vi "Convert Variant to NT Cluster.vi"(11 "NewVal":variant) -> (3 "Field Value":T1)   [LabVIEW 2017]
doc: "Attempt to convert the LV variant type to the various NT types. If not able to do so, it may be stored as a serialized variant or become an invalid NT v ariable."
uses:
  <vilib>/Rock Robotics/Network Tables/Field Data.ctl
  <vilib>/Rock Robotics/Network Tables/Field Type.ctl
  <vilib>/Rock Robotics/Network Tables/Sequence.ctl
panel:
  out "type string":i16[](array[numeric]) format="%.0x"
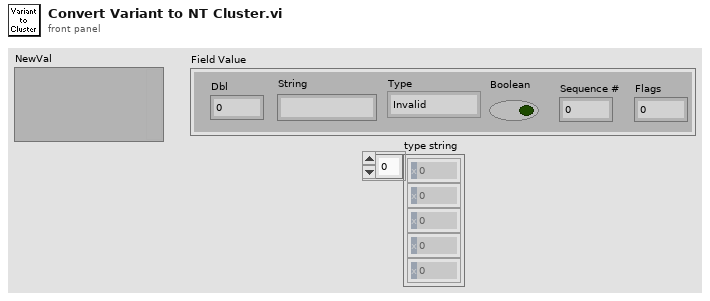
[diagram p1: front panel]
types:
  T1 = typedef "Field Data.ctl" = cluster{"Dbl":dbl, "String":string, "Type":T2, "Boolean":bool, "Sequence #":T3, "Flags":u8}
  T2 = typedef "Field Type.ctl" = enum8{"Invalid", "Bool", "Numeric", "String", "Raw", "Boolean Array", "Numeric Array", "String Array", "RPC"}
  T3 = typedef "Sequence.ctl" = u16
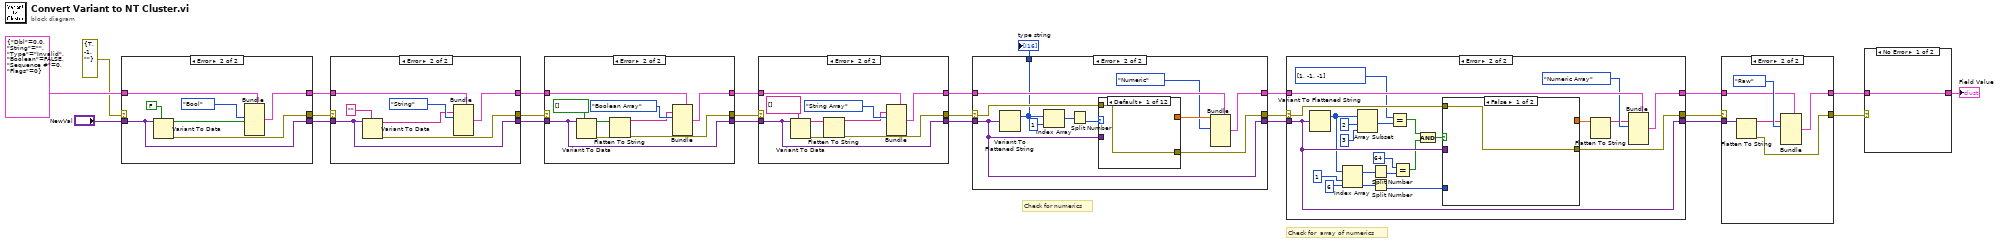
[diagram p0: block diagram]
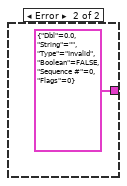
[diagram p3: hidden frame]
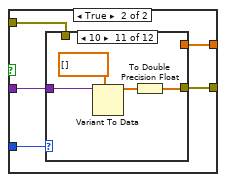
[diagram p5: hidden frame]
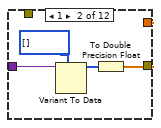
[diagram p7: hidden frame]
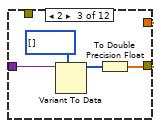
[diagram p8: hidden frame]
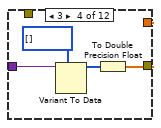
[diagram p9: hidden frame]
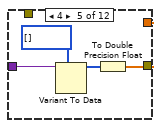
[diagram p10: hidden frame]
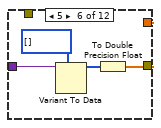
[diagram p11: hidden frame]
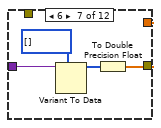
[diagram p12: hidden frame]
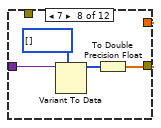
[diagram p13: hidden frame]
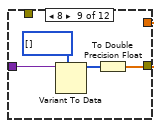
[diagram p14: hidden frame]
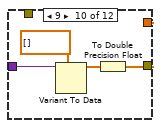
[diagram p15: hidden frame]
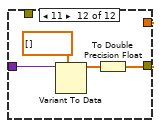
[diagram p16: hidden frame]
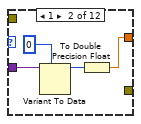
[diagram p18: hidden frame]
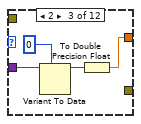
[diagram p19: hidden frame]
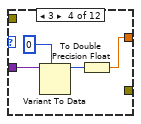
[diagram p20: hidden frame]
diagram:
  # "Check for  array of numerics"
  # "Check for numerics"
  n1 = case shown="Error" errorcluster {"status"=TRUE, "code"=-1, "source"=""} ("error constant") {
    selector: errorcluster {"status"=TRUE, "code"=-1, "source"=""} ("error constant") -> [w27 _]
    tunnel: "NewVal" -> [w26 w31]
    tunnel: T1 {"Dbl"=0.0, "String"="", "Type"=enum."Invalid", "Boolean"=FALSE, "Sequence #"=0, "Flags"=0} ("Field Value") -> [w28 w35]
    tunnel: [w28 w32] -> w19
    tunnel: [w27 w33] -> w18
    tunnel: [w26 w31] -> w17
    frame No Error {
    }
    frame Error {
      n2 = Variant To Data(type=FALSE ("status"), Variant=w31) -> (data=w29:bool, error out=w33:errorcluster)  [unwired: 1 in]
      n3 = Bundle(cluster=w35, "Type"=Field_Type."Bool", "Boolean"=w29) -> (w32:T1)  [unwired: 4 in]
    }
  }
  n4 = case shown="Error" w18 {
    selector: w18 -> [w37 _]
    tunnel: w17 -> [w36 w39]
    tunnel: w19 -> [w38 w44]
    tunnel: [w38 w40] -> w24
    tunnel: [w37 w41] -> w25
    tunnel: [w36 w39] -> w23
    frame No Error {
    }
    frame Error {
      n5 = Variant To Data(type="", Variant=w39) -> (data=w42:string, error out=w41:errorcluster)  [unwired: 1 in]
      n6 = Bundle(cluster=w44, "String"=w42, "Type"=Field_Type."String") -> (w40:T1)  [unwired: 4 in]
    }
  }
  n7 = case shown="Error" w25 {
    selector: w25 -> [w47 _]
    tunnel: w23 -> [w46 w54]
    tunnel: w24 -> [w48 w57]
    tunnel: [w48 w55] -> w22
    tunnel: [w47 w49] -> w21
    tunnel: [w46 w54] -> w20
    frame No Error {
    }
    frame Error {
      n8 = Variant To Data(type=bool[] [], Variant=w54) -> (data=w51:bool[], error out=w52:errorcluster)  [unwired: 1 in]
      n9 = Flatten To String(anything=w51, error in (no error)=w52) -> (data string=w50:string, error out=w49:errorcluster)  [unwired: 2 in, 1 out]
      n10 = Bundle(cluster=w57, "String"=w50, "Type"=Field_Type."Boolean Array") -> (w55:T1)  [unwired: 4 in]
    }
  }
  n11 = case shown="Error" w21 {
    selector: w21 -> [w59 _]
    tunnel: w20 -> [w58 w66]
    tunnel: w22 -> [w60 w69]
    tunnel: [w60 w67] -> w13
    tunnel: [w59 w62] -> w12
    tunnel: [w58 w66] -> w11
    frame No Error {
    }
    frame Error {
      n12 = Variant To Data(type=string[] [], Variant=w66) -> (data=w64:string[], error out=w65:errorcluster)  [unwired: 1 in]
      n13 = Flatten To String(anything=w64, error in (no error)=w65) -> (data string=w63:string, error out=w62:errorcluster)  [unwired: 2 in, 1 out]
      n14 = Bundle(cluster=w69, "String"=w63, "Type"=Field_Type."String Array") -> (w67:T1)  [unwired: 4 in]
    }
  }
  n15 = case shown="Error" w12 {
    selector: w12 -> [w71 w76]
    tunnel: w11 -> [w70 w80]
    tunnel: w13 -> [w72 w83]
    tunnel: [w72 w82] -> w10
    tunnel: [w71 w77] -> w9
    tunnel: [w70 w80] -> w8
    tunnel: [_ w75] -> w6
    frame No Error {
    }
    frame Error {
      n16 = Variant To Flattened String(Variant=w80) -> (1:w75:i16[])  [unwired: 1 out]
      n17 = Index Array(array=w75, index=1) -> (element=w74:i16)
      n18 = Split Number(x=w74) -> (lo(x)=w73:u8)  [unwired: 1 out]
      n19 = case shown="Default" w73 {
        tunnel: w80 -> [_ w88 w92 w96 w100 w104 w108 w112 w116 w120 w124 w128]
        tunnel: [_ w85 w89 w93 w97 w101 w105 w109 w113 w117 w121 w125] -> w79
        tunnel: [w84 _ _ _ _ _ _ _ _ _ _ _] -> w77
        tunnel: w76 -> [w84 _ _ _ _ _ _ _ _ _ _ _]
        frame Default {
        }
        frame 1 {
          n20 = Variant To Data(type=i8 0, Variant=w88) -> (data=w86:i8)  [unwired: 1 in, 1 out]
          n21 = To Double Precision Float(number=w86) -> (double precision float=w85:dbl)
        }
        frame 2 {
          n22 = Variant To Data(type=i16 0, Variant=w92) -> (data=w90:i16)  [unwired: 1 in, 1 out]
          n23 = To Double Precision Float(number=w90) -> (double precision float=w89:dbl)
        }
        frame 3 {
          n24 = Variant To Data(type=0, Variant=w96) -> (data=w94:i32)  [unwired: 1 in, 1 out]
          n25 = To Double Precision Float(number=w94) -> (double precision float=w93:dbl)
        }
        frame 4 {
          n26 = Variant To Data(type=i64 0, Variant=w100) -> (data=w98:i64)  [unwired: 1 in, 1 out]
          n27 = To Double Precision Float(number=w98) -> (double precision float=w97:dbl)
        }
        frame 5 {
          n28 = Variant To Data(type=u8 0, Variant=w104) -> (data=w102:u8)  [unwired: 1 in, 1 out]
          n29 = To Double Precision Float(number=w102) -> (double precision float=w101:dbl)
        }
        frame 6 {
          n30 = Variant To Data(type=u16 0, Variant=w108) -> (data=w106:u16)  [unwired: 1 in, 1 out]
          n31 = To Double Precision Float(number=w106) -> (double precision float=w105:dbl)
        }
        frame 7 {
          n32 = Variant To Data(type=u32 0, Variant=w112) -> (data=w110:u32)  [unwired: 1 in, 1 out]
          n33 = To Double Precision Float(number=w110) -> (double precision float=w109:dbl)
        }
        frame 8 {
          n34 = Variant To Data(type=u64 0, Variant=w116) -> (data=w114:u64)  [unwired: 1 in, 1 out]
          n35 = To Double Precision Float(number=w114) -> (double precision float=w113:dbl)
        }
        frame 9 {
          n36 = Variant To Data(type=sgl 0.0, Variant=w120) -> (data=w118:sgl)  [unwired: 1 in, 1 out]
          n37 = To Double Precision Float(number=w118) -> (double precision float=w117:dbl)
        }
        frame 10 {
          n38 = Variant To Data(type=0.0, Variant=w124) -> (data=w122:dbl)  [unwired: 1 in, 1 out]
          n39 = To Double Precision Float(number=w122) -> (double precision float=w121:dbl)
        }
        frame 11 {
          n40 = Variant To Data(type=ext 0.0, Variant=w128) -> (data=w126:ext)  [unwired: 1 in, 1 out]
          n41 = To Double Precision Float(number=w126) -> (double precision float=w125:dbl)
        }
      }
      n42 = Bundle(cluster=w83, "Dbl"=w79, "Type"=Field_Type."Numeric") -> (w82:T1)  [unwired: 4 in]
    }
  }
  "type string" <- w6
  n43 = case shown="Error" w9 {
    selector: w9 -> [w130 w148]
    tunnel: w8 -> [w129 w151]
    tunnel: w10 -> [w131 w154]
    tunnel: [w131 w153] -> w5
    tunnel: [w130 w149] -> w3
    tunnel: [w129 w151] -> w4
    frame No Error {
    }
    frame Error {
      n44 = Variant To Flattened String(Variant=w151) -> (1:w144:i16[])  [unwired: 1 out]
      n45 = Index Array(array=w144, index #1=1 ("index"), index #2=6 ("index")) -> (element #1=w137:i16, element #2=w140:i16)
      n46 = Array Subset(array=w144, index=2, length=3 ("index")) -> (w146:i16[])
      n47 = Split Number(x=w137) -> (lo(x)=w136:u8)  [unwired: 1 out]
      n48 = Split Number(x=w140) -> (lo(x)=w139:u8)  [unwired: 1 out]
      n49 = Equal?(x=i16[] [1, -1, -1], y=w146) -> (x = y?=w133:bool)
      n50 = Equal?(x=i16 64 ("index"), y=w136) -> (x = y?=w132:bool)
      n51 = And(x=w133, y=w132) -> (x .and. y?=w134:bool)
      n52 = case shown="False" w134 {
        tunnel: w151 -> [_ w160]
        tunnel: [_ w159] -> w143
        tunnel: [w155 w158] -> w149
        tunnel: w148 -> [w155 w157]
        tunnel: w139 -> [_ w156]
        frame False {
        }
        frame True {
          n53 = case shown="10" w156 {
            tunnel: w160 -> [_ w165 w169 w173 w177 w181 w185 w189 w193 w197 w201 w205]
            tunnel: [_ w162 w167 w171 w175 w179 w183 w187 w191 w195 w199 w203] -> w159
            tunnel: [w161 _ _ _ _ _ _ _ _ _ _ _] -> w158
            tunnel: w157 -> [w161 _ _ _ _ _ _ _ _ _ _ _]
            frame Default {
            }
            frame 1 {
              n54 = Variant To Data(type=i8[] [], Variant=w165) -> (data=w164:i8[])  [unwired: 1 in, 1 out]
              n55 = To Double Precision Float(number=w164) -> (double precision float=w162:dbl[])
            }
            frame 2 {
              n56 = Variant To Data(type=i16[] [], Variant=w169) -> (data=w168:i16[])  [unwired: 1 in, 1 out]
              n57 = To Double Precision Float(number=w168) -> (double precision float=w167:dbl[])
            }
            frame 3 {
              n58 = Variant To Data(type=i32[] [], Variant=w173) -> (data=w172:i32[])  [unwired: 1 in, 1 out]
              n59 = To Double Precision Float(number=w172) -> (double precision float=w171:dbl[])
            }
            frame 4 {
              n60 = Variant To Data(type=i64[] [], Variant=w177) -> (data=w176:i64[])  [unwired: 1 in, 1 out]
              n61 = To Double Precision Float(number=w176) -> (double precision float=w175:dbl[])
            }
            frame 5 {
              n62 = Variant To Data(type=u8[] [], Variant=w181) -> (data=w180:u8[])  [unwired: 1 in, 1 out]
              n63 = To Double Precision Float(number=w180) -> (double precision float=w179:dbl[])
            }
            frame 6 {
              n64 = Variant To Data(type=u16[] [], Variant=w185) -> (data=w184:u16[])  [unwired: 1 in, 1 out]
              n65 = To Double Precision Float(number=w184) -> (double precision float=w183:dbl[])
            }
            frame 7 {
              n66 = Variant To Data(type=u32[] [], Variant=w189) -> (data=w188:u32[])  [unwired: 1 in, 1 out]
              n67 = To Double Precision Float(number=w188) -> (double precision float=w187:dbl[])
            }
            frame 8 {
              n68 = Variant To Data(type=u64[] [], Variant=w193) -> (data=w192:u64[])  [unwired: 1 in, 1 out]
              n69 = To Double Precision Float(number=w192) -> (double precision float=w191:dbl[])
            }
            frame 9 {
              n70 = Variant To Data(type=sgl[] [], Variant=w197) -> (data=w196:sgl[])  [unwired: 1 in, 1 out]
              n71 = To Double Precision Float(number=w196) -> (double precision float=w195:dbl[])
            }
            frame 10 {
              n72 = Variant To Data(type=dbl[] [], Variant=w201) -> (data=w200:dbl[])  [unwired: 1 in, 1 out]
              n73 = To Double Precision Float(number=w200) -> (double precision float=w199:dbl[])
            }
            frame 11 {
              n74 = Variant To Data(type=ext[] [], Variant=w205) -> (data=w204:ext[])  [unwired: 1 in, 1 out]
              n75 = To Double Precision Float(number=w204) -> (double precision float=w203:dbl[])
            }
          }
        }
      }
      n76 = Flatten To String(anything=w143) -> (data string=w142:string)  [unwired: 3 in, 2 out]
      n77 = Bundle(cluster=w154, "String"=w142, "Type"=Field_Type."Numeric Array") -> (w153:T1)  [unwired: 4 in]
    }
  }
  n78 = case shown="Error" w3 {
    selector: w3 -> [w207 _]
    tunnel: w5 -> [w206 w212]
    tunnel: w4 -> [_ w210]
    tunnel: [w207 w208] -> w2
    tunnel: [w206 w209] -> w1
    frame No Error {
    }
    frame Error {
      n79 = Flatten To String(anything=w210) -> (data string=w211:string, error out=w208:errorcluster)  [unwired: 3 in, 1 out]
      n80 = Bundle(cluster=w212, "String"=w211, "Type"=Field_Type."Raw") -> (w209:T1)  [unwired: 4 in]
    }
  }
  n81 = case shown="No Error" w2 {
    tunnel: w1 -> [w214 _]
    tunnel: [w214 T1 {"Dbl"=0.0, "String"="", "Type"=enum."Invalid", "Boolean"=FALSE, "Sequence #"=0, "Flags"=0} ("Field Value")] -> w7
    frame No Error {
    }
    frame Error {
    }
  }
  "Field Value" <- w7
